vi "Aggiorna collaudo con nuovo file taratura.vi"(8 "Densità per ricalcolo P2":dbl, 9 "rpm nom":dbl, 10 "Array in":string[][](array[string]), 11 "COEFF":T1) -> (2 "Array in out":string[][](array[string]))   [LabVIEW 2019]
uses:
  TypeDef/Indici.ctl
  <vilib>/Utility/file.llb/Read Delimited Spreadsheet (string).vi
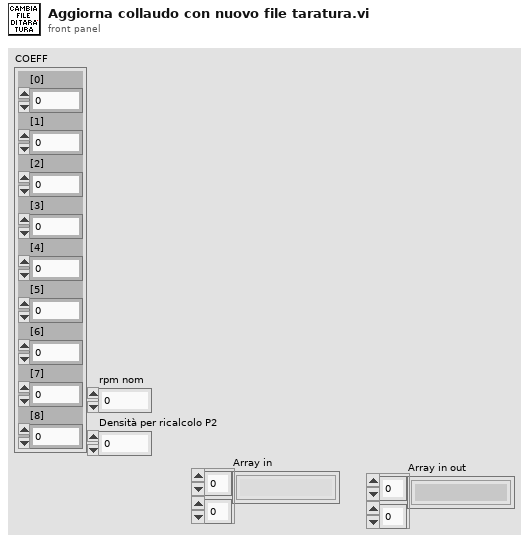
[diagram p1: front panel]
types:
  T1 = cluster{"[0]":dbl, "[1]":dbl, "[2]":dbl, "[3]":dbl, "[4]":dbl, "[5]":dbl, "[6]":dbl, "[7]":dbl, "[8]":dbl}
  T2 = cluster{"Af":dbl, "Bf":dbl, "Cf":dbl, "Df":dbl, "Ef":dbl, "Ff":dbl, "Gf":dbl, "Hf":dbl, "Jf":dbl, "Kf":dbl, "If":dbl, "Ar":dbl, "Br":dbl, "Cr":dbl, "Dr":dbl, "Er":dbl, "Fr":dbl, "Gr":dbl, "Hr":dbl, "Jr":dbl, "Kr":dbl, "Ir":dbl}
  T3 = typedef "Indici.ctl" = cluster{"Q":i32, "Htot":i32, "NPSH":i32, "P3":i32, "etap":i32, "temperature":cluster{"DT":i32, "DTmarcia":i32, "DTaux":i32, "TC1":i32, "TC2":i32, "TC3":i32, "TC4":i32}, "tempo":i32, "P2":i32, "P1":i32, "etaGr":i32, "RPM":i32}
  T4 = cluster{"P1":i32, "P2":i32, "P3":i32, "Eta motore":i32, "Eta pompa":i32}
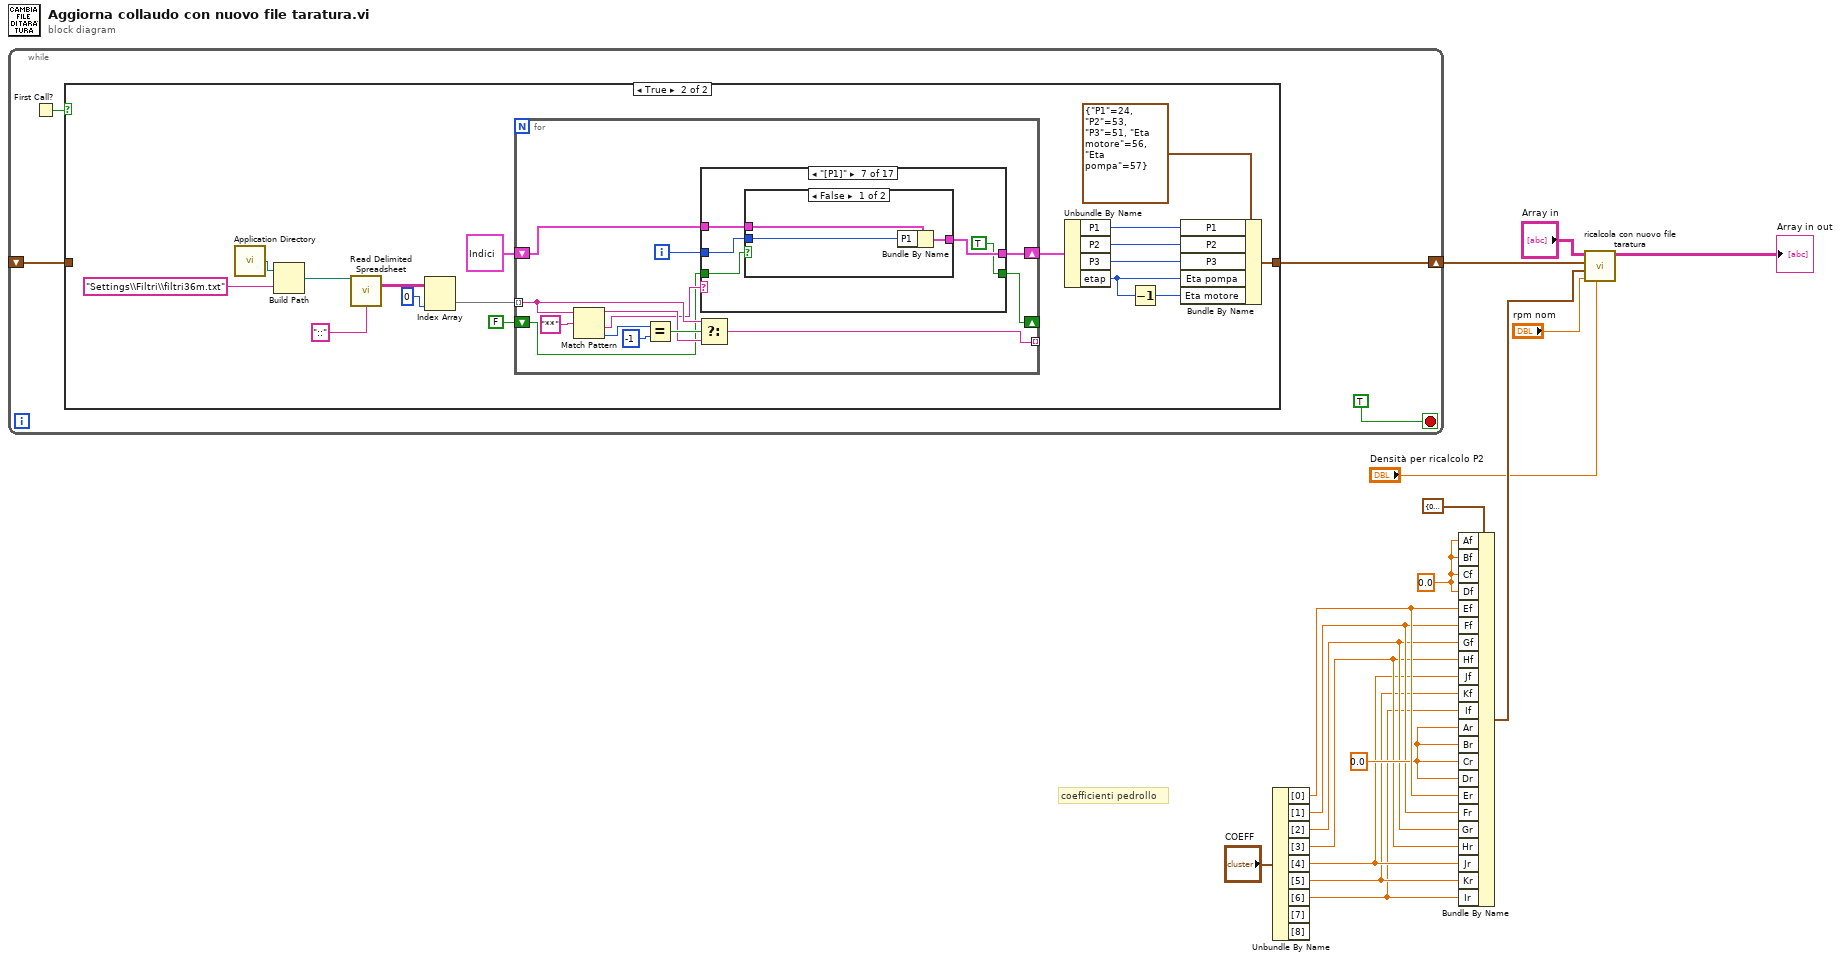
[diagram p0: block diagram]
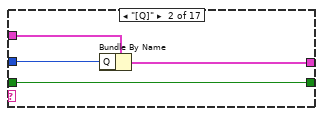
[diagram p4: hidden frame]
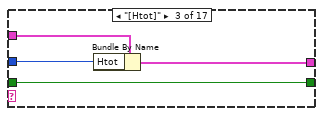
[diagram p5: hidden frame]
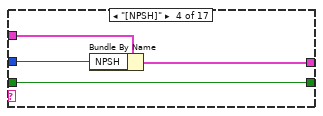
[diagram p6: hidden frame]
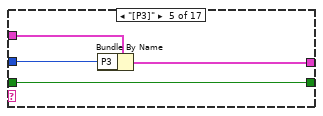
[diagram p7: hidden frame]
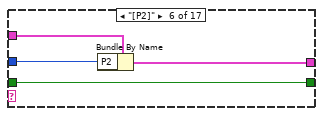
[diagram p8: hidden frame]
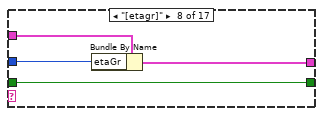
[diagram p10: hidden frame]
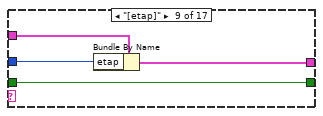
[diagram p11: hidden frame]
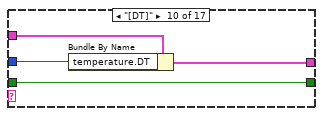
[diagram p12: hidden frame]
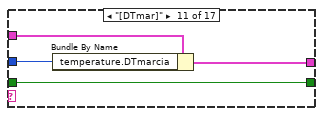
[diagram p13: hidden frame]
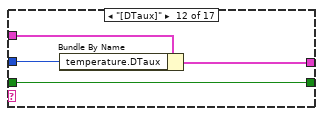
[diagram p14: hidden frame]
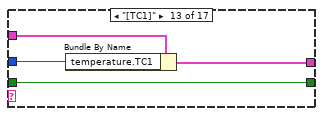
[diagram p15: hidden frame]
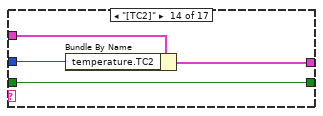
[diagram p16: hidden frame]
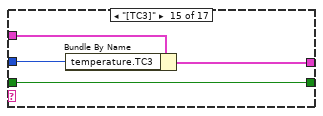
[diagram p17: hidden frame]
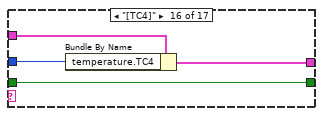
[diagram p18: hidden frame]
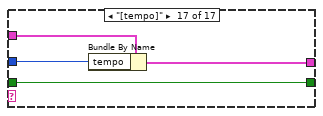
[diagram p19: hidden frame]
diagram:
  w13 = 0.0 ("Er")
  w17 = 0.0 ("Ef")
  # "coefficienti pedrollo"
  n1 = while {
    shift-right: [w20] -> w1
    shift-left: _ -> [w19]
    stop <- TRUE stop-if-true
    n2 = First Call?() -> (First Call?: T/F=w18:bool)
    n3 = case shown="True" w18 {
      tunnel: [w22 w23] -> w20
      tunnel: w19 -> [w22 _]
      frame False {
      }
      frame True {
        n4 = call <vilib>:"Application Directory.vi"() -> ("Application Directory"=w39:path)
        n5 = Build Path(base path=w39, name or relative path="Settings\\Filtri\\filtri36m.txt") -> (appended path=w37:path)
        n6 = call-poly <vilib>:"Read Delimited Spreadsheet.vi"("file path (dialog if empty)"=w37, "delimiter (\\t)"="::" ("delimiter (\\t)")) -> ("all rows"=w35:string[][])  [unwired: 8 in, 5 out]
        n7 = Index Array(array=w35, index (col)=0 ("disabled index (col)")) -> (element=w33:string[])  [unwired: 1 in]
        n8 = for {
          tunnel: w33 -> [w46] mode=indexing
          tunnel: [w47] -> _ mode=indexing
          shift-right: [w43] -> w31
          shift-left: T3 {"Q"=0, "Htot"=0, "NPSH"=0, "P3"=0, "etap"=0, "temperature"={"DT"=0, "DTmarcia"=0, "DTaux"=0, "TC1"=0, "TC2"=0, "TC3"=0, "TC4"=0}, "tempo"=0, "P2"=0, "P1"=0, "etaGr"=0, "RPM"=0} -> [w44]
          shift-right: [w41] -> _
          shift-left: FALSE -> [w40]
          i -> [w42]
          n9 = Match Pattern(string=w46, regular expression="**") -> (before substring=w48:string, after substring=w45:string, offset past match=w51:i32)  [unwired: 1 in, 1 out]
          n10 = Equal?(x=w51, y=-1) -> (x = y?=w49:bool)
          n11 = Select(t=w46, s=w49, f=w48) -> (s? t:f=w47:string)
          n12 = case shown="\"[P1]\"" w45 {
            tunnel: w44 -> [w54 w58 w62 w66 w70 w74 w79 w87 w91 w95 w99 w103 w107 w111 w115 w119 w123]
            tunnel: [w54 w57 w60 w65 w68 w73 w78 w86 w89 w94 w98 w102 w106 w110 w114 w118 w122] -> w43
            tunnel: w42 -> [_ w56 w61 w64 w69 w72 w77 w85 w90 w93 w97 w101 w105 w109 w113 w117 w121]
            tunnel: [w53 w55 w59 w63 w67 w71 TRUE w84 w88 w92 w96 w100 w104 w108 w112 w116 w120] -> w41
            tunnel: w40 -> [w53 w55 w59 w63 w67 w71 w75 w84 w88 w92 w96 w100 w104 w108 w112 w116 w120]
            frame "False", Default {
            }
            frame "[Q]" {
              n13 = Bundle By Name(cluster=w58, "Q"=w56) -> (w57:T3)
            }
            frame "[Htot]" {
              n14 = Bundle By Name(cluster=w62, "Htot"=w61) -> (w60:T3)
            }
            frame "[NPSH]" {
              n15 = Bundle By Name(cluster=w66, "NPSH"=w64) -> (w65:T3)
            }
            frame "[P3]" {
              n16 = Bundle By Name(cluster=w70, "P3"=w69) -> (w68:T3)
            }
            frame "[P2]" {
              n17 = Bundle By Name(cluster=w74, "P2"=w72) -> (w73:T3)
            }
            frame "[P1]" {
              n18 = case shown="False" w75 {
                tunnel: w79 -> [w82 w83]
                tunnel: [w81 w83] -> w78
                tunnel: w77 -> [w80 _]
                frame False {
                  n19 = Bundle By Name(cluster=w82, "P1"=w80) -> (w81:T3)
                }
                frame True {
                }
              }
            }
            frame "[etagr]" {
              n20 = Bundle By Name(cluster=w87, "etaGr"=w85) -> (w86:T3)
            }
            frame "[etap]" {
              n21 = Bundle By Name(cluster=w91, "etap"=w90) -> (w89:T3)
            }
            frame "[DT]" {
              n22 = Bundle By Name(cluster=w95, "temperature.DT"=w93) -> (w94:T3)
            }
            frame "[DTmar]" {
              n23 = Bundle By Name(cluster=w99, "temperature.DTmarcia"=w97) -> (w98:T3)
            }
            frame "[DTaux]" {
              n24 = Bundle By Name(cluster=w103, "temperature.DTaux"=w101) -> (w102:T3)
            }
            frame "[TC1]" {
              n25 = Bundle By Name(cluster=w107, "temperature.TC1"=w105) -> (w106:T3)
            }
            frame "[TC2]" {
              n26 = Bundle By Name(cluster=w111, "temperature.TC2"=w109) -> (w110:T3)
            }
            frame "[TC3]" {
              n27 = Bundle By Name(cluster=w115, "temperature.TC3"=w113) -> (w114:T3)
            }
            frame "[TC4]" {
              n28 = Bundle By Name(cluster=w119, "temperature.TC4"=w117) -> (w118:T3)
            }
            frame "[tempo]" {
              n29 = Bundle By Name(cluster=w123, "tempo"=w121) -> (w122:T3)
            }
          }
        }
        n30 = Unbundle By Name(w31) -> ("P1"=w30:i32, "P2"=w29:i32, "P3"=w28:i32, "etap"=w26:i32)
        n31 = Decrement(x=w26) -> (x-1=w25:i32)
        n32 = Bundle By Name(cluster=T4 {"P1"=24, "P2"=53, "P3"=51, "Eta motore"=56, "Eta pompa"=57} ("Indici"), "P1"=w30, "P2"=w29, "P3"=w28, "Eta pompa"=w26, "Eta motore"=w25) -> (w23:T4)
      }
    }
  }
  n33 = Unbundle By Name("COEFF") -> ("[0]"=w14:dbl, "[1]"=w12:dbl, "[2]"=w11:dbl, "[3]"=w10:dbl, "[4]"=w9:dbl, "[5]"=w8:dbl, "[6]"=w7:dbl)  [unwired: 2 out]
  n34 = Bundle By Name(cluster=T2 {"Af"=0.0, "Bf"=0.0, "Cf"=0.0, "Df"=0.0, "Ef"=0.0, "Ff"=0.0, "Gf"=0.0, "Hf"=0.0, "Jf"=0.0, "Kf"=0.0, "If"=0.0, "Ar"=0.0, "Br"=0.0, "Cr"=0.0, "Dr"=0.0, "Er"=0.0, "Fr"=0.0, "Gr"=0.0, "Hr"=0.0, "Jr"=0.0, "Kr"=0.0, "Ir"=0.0} ("Coefficenti P2"), "Af"=w17, "Bf"=w17, "Cf"=w17, "Df"=w17, "Ef"=w14, "Ff"=w12, "Gf"=w11, "Hf"=w10, "Jf"=w9, "Kf"=w8, "If"=w7, "Ar"=w13, "Br"=w13, "Cr"=w13, "Dr"=w13, "Er"=w14, "Fr"=w12, "Gr"=w11, "Hr"=w10, "Jr"=w9, "Kr"=w8, "Ir"=w7) -> (w6:T2)
  n35 = call "ricalcola con nuovo file taratura.vi"("Densità per ricalcolo P2"="Densità per ricalcolo P2", "rpm nom"="rpm nom", "Coefficenti P2"=w6, "Indici"=w1, "dati in"="Array in") -> ("dati out"=→"Array in out":string[][])  [unwired: 6 in]
